vi "Plot Editor.vi"(6 "Original Plot Idx":i32=-1, 7 "Original Graph Name":string, 8 "Error In":errorcluster, 9 "Plot Style in":T2={"Plot Index"=0, "Plot.Bar Plot Style"=0, "Plot.DigitalLineStyle"=1, "Plot.TransitionLocation"=2, "Plot.Transition Type"=0, "Plot.Fill To"=-1, "Plot.Fill/Pt. Color"=16777222, "Plot.Label Format"=3, "Plot.Line Style"=0, "Plot.Line Width"=1, "Plot.Plot Color"=16777222, "Plot.Plot Interpolation"=2, "Plot.Plot Name"="", "Plot.Point Style"=0, "Plot.Visible?"=TRUE, "Plot.XScaleIdx"=0, "Plot.YScaleIdx"=0, "Plot.Anti-aliased"=TRUE}, 10 "Plot in":T3, 11 "Original Graph Refnum":T1) -> (0 "Error Out":errorcluster, 1 "Plot Style out":T2, 2 "Plot out":T3)   [LabVIEW 2019, in "Plot Editor.lvlib"]
uses:
  Plot Editor.lvlib
  XY Graph Plot Properties.ctl
  XY Plot Data.ctl
  XY Graph Refnum.ctl
  Plot Editor Q [Element].ctl
  Plot Editor Q [Event] List.ctl
  Plot Editor Internal Variables.ctl
  <vilib>/Utility/error.llb/DialogType.ctl
  <vilib>/Utility/miscctls.llb/LVPoint32TypeDef.ctl
  XY Graph Add-Ons.lvlib
  Notebook.lvlib
  Define Ramp Array Dialog.vi
  Rich Text Box.lvlib
  Variant to Data.lvlib
panel:
  in  "X Array":dbl[](array[numeric])
  in  "Copy":bool
  in  "Cancel":bool
  out "Error":errorcluster
  in  "Reset Style":bool
  out "Y Array Size":i32
  in  "Cancel Data Edit":bool
  in  "OK":bool
  out "X Array Size":i32
  in  "Y Array":dbl[](array[numeric]) caption="X Array"
  out "Plot Preview":cluster{"X Array":dbl[], "Y Array":dbl[]}[](graph)
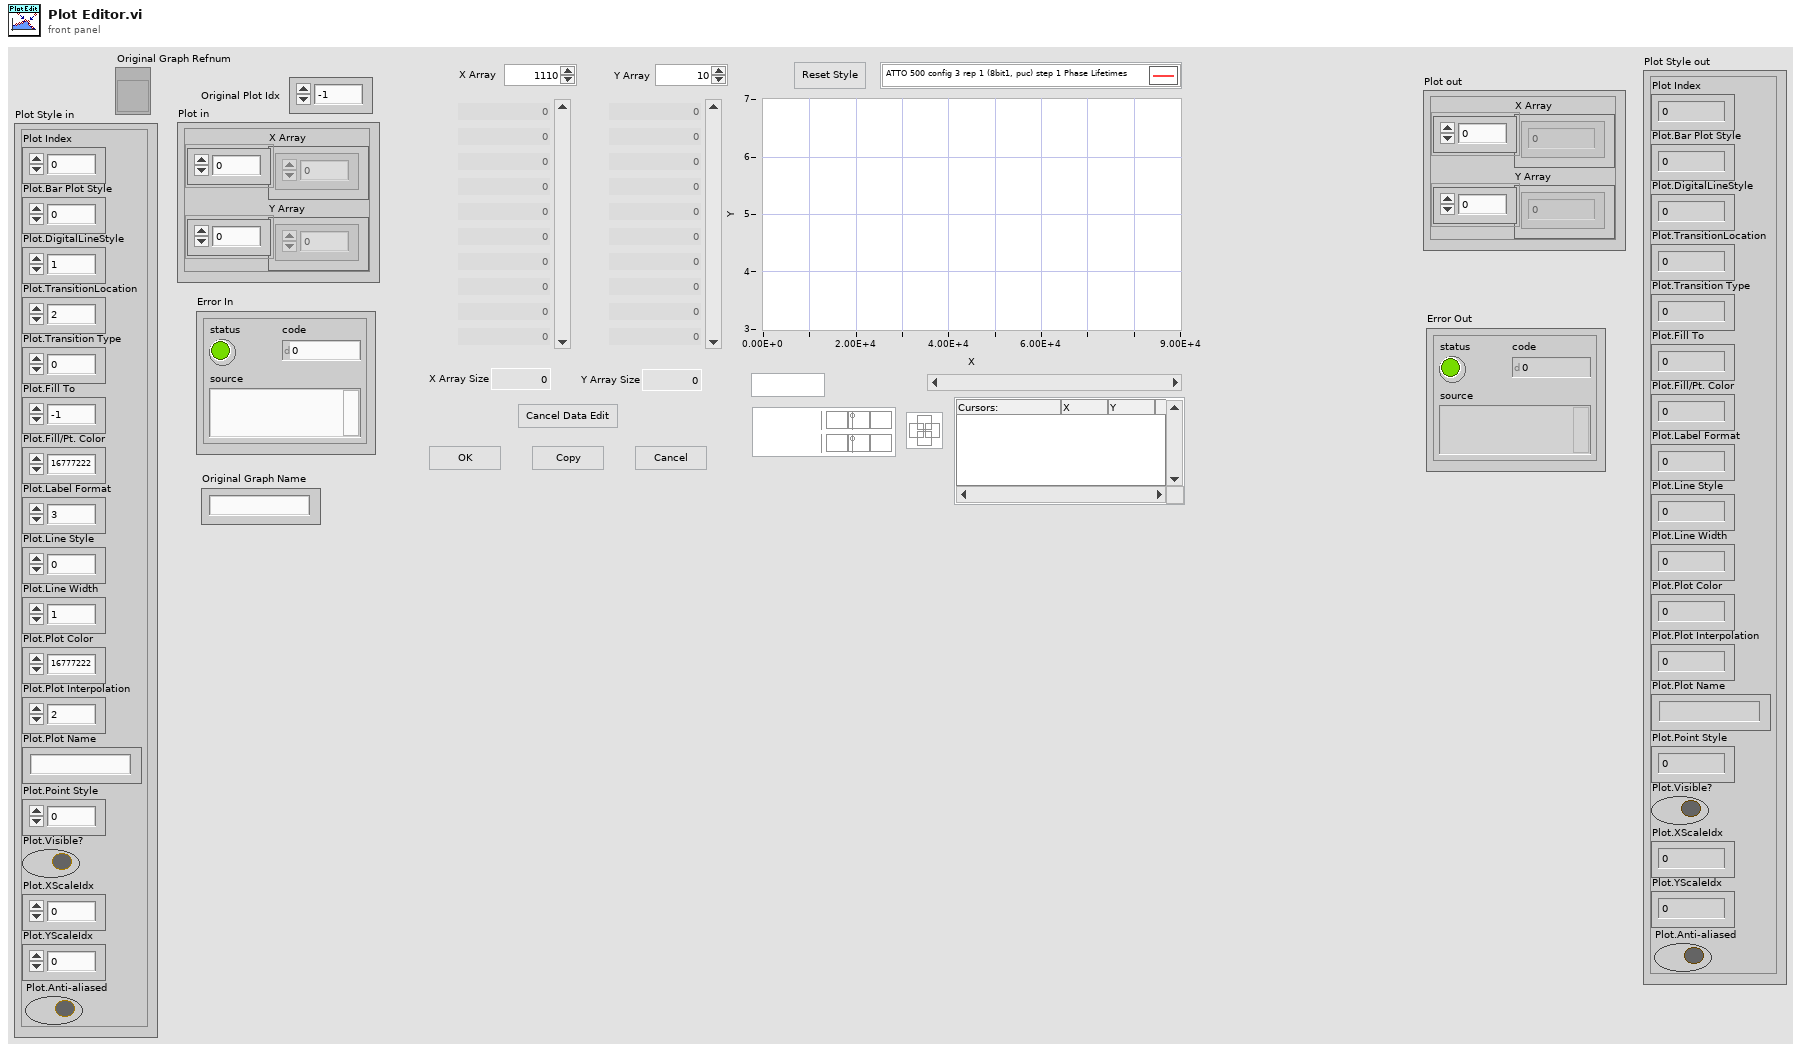
[diagram p1: front panel]
types:
  T1 = typedef "XY Graph Add-Ons.lvlib/XY Graph Refnum.ctl" = refnum<vi>
  T2 = typedef "XY Graph Plot Properties.ctl" = cluster{"Plot Index":i32, "Plot.Bar Plot Style":u8, "Plot.DigitalLineStyle":u8, "Plot.TransitionLocation":u8, "Plot.Transition Type":u8, "Plot.Fill To":i16, "Plot.Fill/Pt. Color":u32, "Plot.Label Format":u8, "Plot.Line Style":u8, "Plot.Line Width":u8, "Plot.Plot Color":u32, "Plot.Plot Interpolation":u8, "Plot.Plot Name":string, "Plot.Point Style":u8, "Plot.Visible?":bool, "Plot.XScaleIdx":u32, "Plot.YScaleIdx":u32, "Plot.Anti-aliased":bool}
  T3 = typedef "XY Plot Data.ctl" = cluster{"X Array":dbl[], "Y Array":dbl[]}
  T4 = typedef "Plot Editor.lvlib/Plot Editor Q [Element].ctl" = cluster{"Plot Editor Q Event":T5, "Data":variant}
  T5 = typedef "Plot Editor.lvlib/Plot Editor Q [Event] List.ctl" = enum16{"Idle", "Initialization", "Controls >> Store", "Store >> Plot", "Update Plot Style", "Check Data Array Alignment", "Reset Data", "Reset Style", "Accept & Quit", "Copy & Quit", "Save Plot", "Load Plot", "Remove out-of-bound Values", "Delete Element", "Insert Element Before", "Insert Element After", "Update output string", "Remove NaN-containing Pairs", "Fill Array with Ramp", "Quit"}
  T6 = typedef "Plot Editor.lvlib/Plot Editor Internal Variables.ctl" = cluster{"X Array":dbl[], "Y Array":dbl[], "XY Plot Properties":T2, "X Array Index Values":u32[], "Y Array Index Values":u32[], "Original XY Plot Properties":T2, "Original X Array":dbl[], "Original Y Array":dbl[], "VI title suffix":string, "Refnum based call":bool}
  T7 = typedef "LVPoint32TypeDef.ctl" = cluster{"Horizontal":i32, "Vertical":i32}
  T8 = typedef "Rich Text Box.lvlib/Text Formatting.ctl" = cluster{"Font":string, "Text Color":T9, "Text Background Color":T9, "Text Style":enum16{"Regular", "Bold", "Italic", "Underline", "Strikeout"}, "Font Size (Points)":dbl, "Text Alignment":i32}
  T9 = typedef "Rich Text Box.lvlib/Text Colors.ctl" = enum16{"Unchanged", "Black", "Blue", "Gray", "Green", "Red", "White"}
  T10 = typedef "DialogType.ctl" = u16
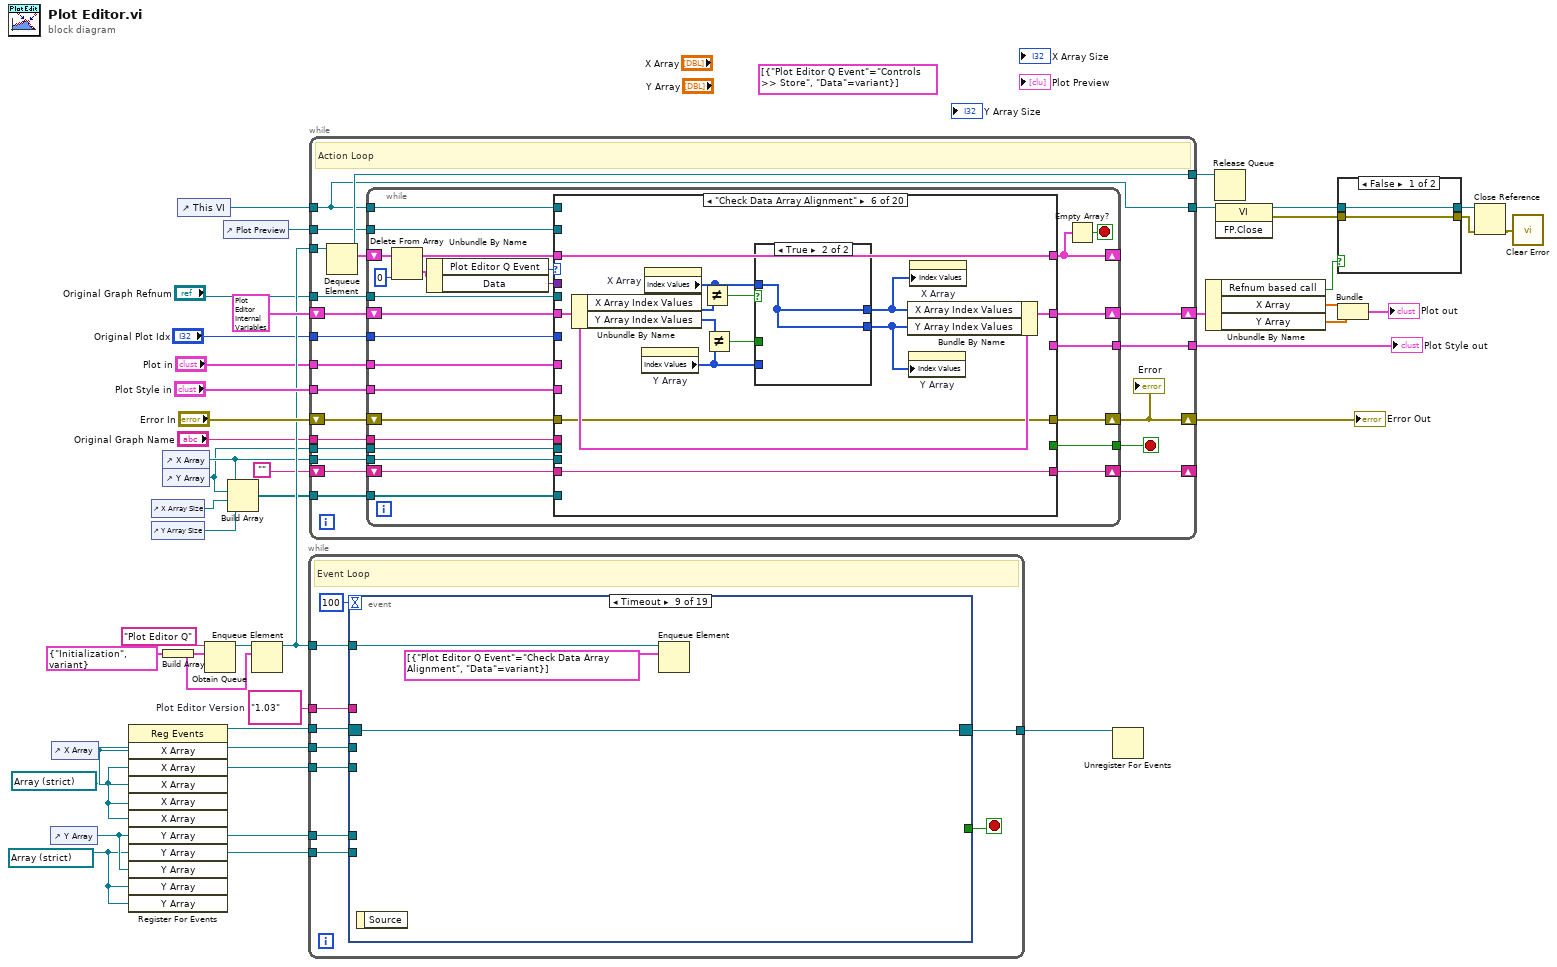
[diagram p0: block diagram]
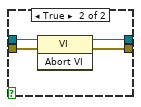
[diagram p2: hidden frame]
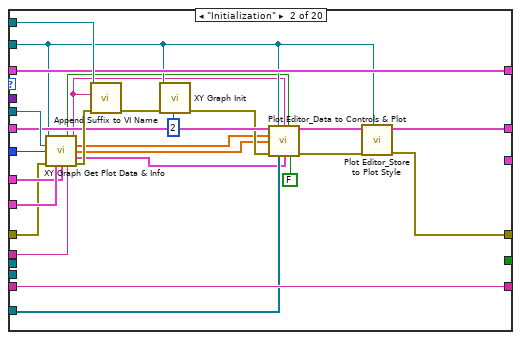
[diagram p4: hidden frame]
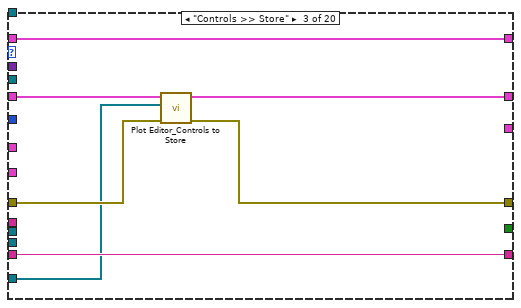
[diagram p5: hidden frame]
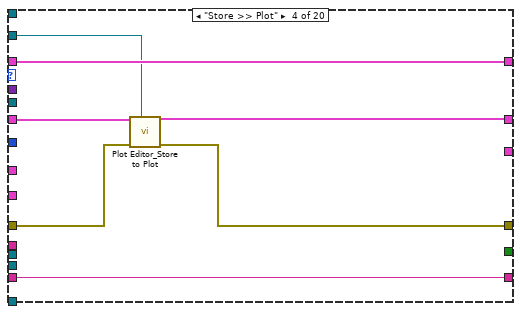
[diagram p6: hidden frame]
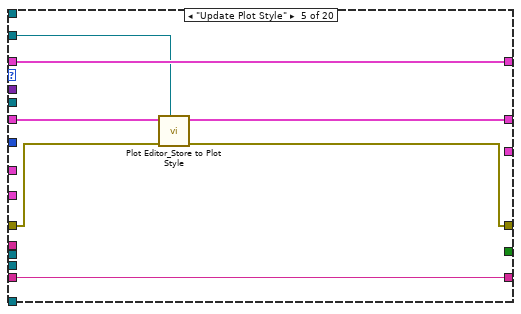
[diagram p7: hidden frame]
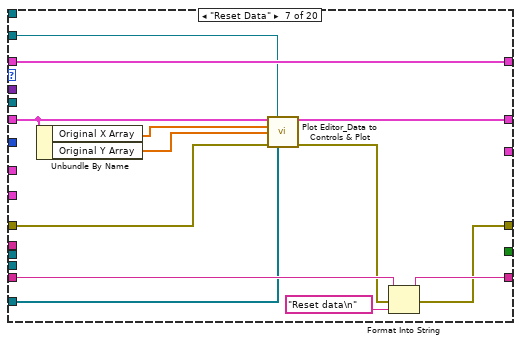
[diagram p10: hidden frame]
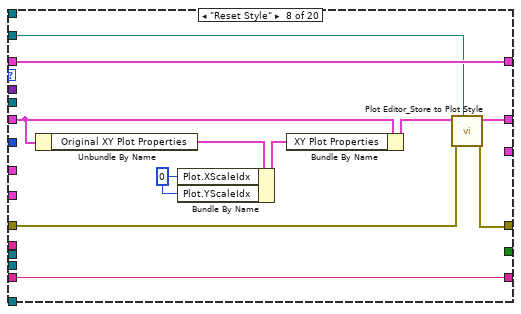
[diagram p11: hidden frame]
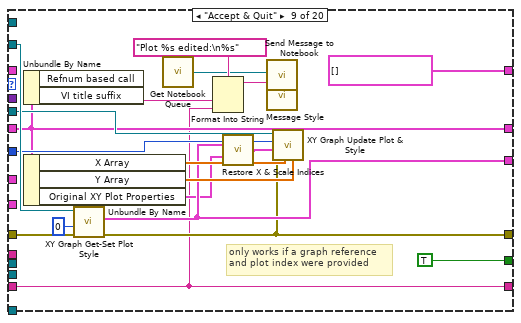
[diagram p12: hidden frame]
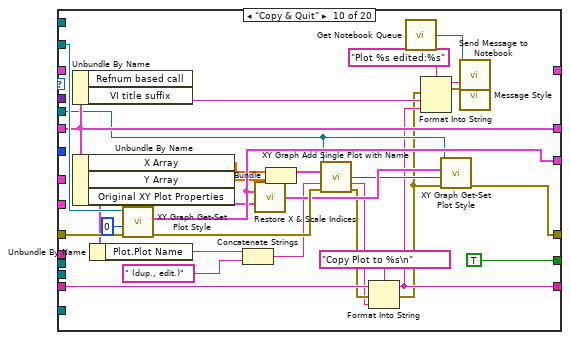
[diagram p13: hidden frame]
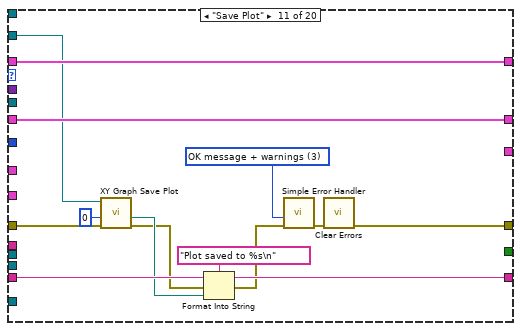
[diagram p14: hidden frame]
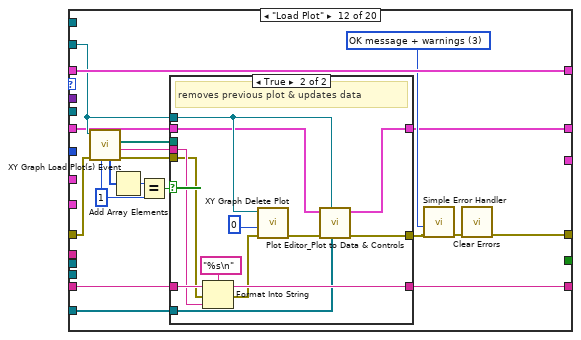
[diagram p15: hidden frame]
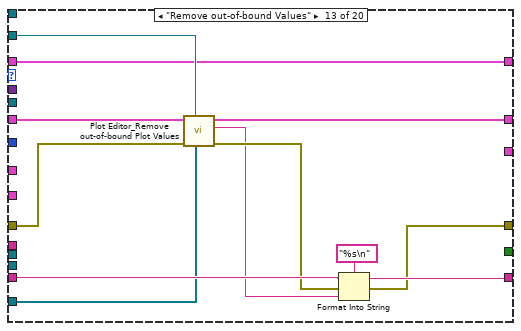
[diagram p17: hidden frame]
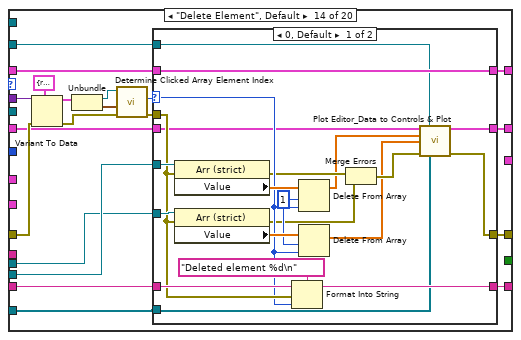
[diagram p18: hidden frame]
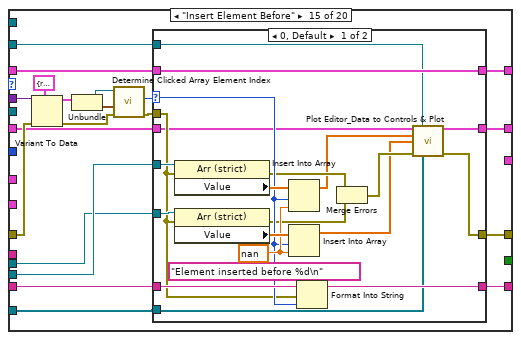
[diagram p20: hidden frame]
diagram:
  w2 = refnum<vi> refnum ("Y Array")
  w1 = refnum<vi> refnum ("X Array")
  (unwired) T4[] [{"Plot Editor Q Event"=enum."Controls >> Store", "Data"=variant}] ("array")
  w25 = "1.03"  # Plot Editor Version
  n1 = control-ref of="Y Array"() -> (w3:refnum<vi>)
  n2 = control-ref of="X Array"() -> (w4:refnum<vi>)
  n3 = register-events(w4, w1, w4, w1, w1, w3, w2, w3, w2, w2) -> (reference out=w24:refnum<event-registration>)  [unwired: 2 in, 1 out]
  n4 = control-ref of="X Array Size"() -> (w7:refnum<vi>)
  n5 = control-ref of="Y Array Size"() -> (w6:refnum<vi>)
  n6 = control-ref of="X Array"() -> (w9:refnum<vi>)
  n7 = control-ref of="Y Array"() -> (w8:refnum<vi>)
  n8 = Build Array(T4 {"Plot Editor Q Event"=enum."Initialization", "Data"=variant} ("Plot Editor Q Element")) -> (w26:T4[])
  n9 = control-ref of="This VI"() -> (w16:refnum<vi>)
  n10 = Obtain Queue(name (unnamed)="Plot Editor Q", element data type=w26) -> (queue out=w39:refnum<queue>)  [unwired: 3 in, 2 out]
  n11 = control-ref of="Plot Preview"() -> (w34:refnum<vi>)
  n12 = Build Array(w9, w8, w7, w6) -> (w5:refnum<vi>[])
  n13 = Enqueue Element(queue=w39, element=w26) -> (queue out=w27:refnum<queue>)  [unwired: 2 in, 2 out]
  n14 = while {
    tunnel: w27 -> [w50]
    tunnel: w25 -> [w49]
    tunnel: w24 -> [w48]
    tunnel: w4 -> [w47]
    tunnel: w3 -> [w46]
    tunnel: [w45] -> w23
    tunnel: w1 -> [w44]
    tunnel: w2 -> [w43]
    stop <- w51 stop-if-true
    # "Event Loop"
    n15 = event shown="[8] Timeout" {
      selector: w48 -> [_ _ _ _ _ w157 w161 w164 w167 w173 w179 w183 w188 _ _ _ _ _ _]
      dyn-events: [_ _ _ _ _ w156 w160 w164 w167 w172 w178 w182 w187 _ _ _ _ _ _] -> w45
      timeout: 100 -> [_ _ _ _ _ _ _ _ _ _ _ _ _ _ _ _ _ _ _]
      tunnel: [w54 w56 _ _ _ _ _ _ _ _ _ _ _ _ _ _ TRUE ("Discard?") TRUE ("Discard?") TRUE ("Discard?")] -> w51
      tunnel: w50 -> [w53 w57 w91 w122 w146 _ _ w163 w166 w169 w174 _ _ w198 w200 w202 w205 w208 w211]
      tunnel: w49 -> [_ w55 _ _ _ _ _ _ _ _ _ _ _ _ _ _ _ _ _]
      tunnel: w47 -> [_ _ _ _ _ w155 _ _ _ w171 _ w181 w186 _ _ _ _ _ _]
      tunnel: w46 -> [_ _ _ _ _ _ w159 _ _ _ w176 _ w185 _ _ _ _ _ _]
      tunnel: w44 -> [_ _ _ _ _ w154 _ _ _ w170 _ w180 _ _ _ _ _ _ _]
      tunnel: w43 -> [_ _ _ _ _ _ w158 _ _ _ w177 _ w184 _ _ _ _ _ _]
      event Panel Close? {
        w54 = TRUE ("Discard?")
        n16 = event-data() -> ()  [unwired: 1 in, 1 out]
        n17 = Enqueue Element(queue=w53, element=T4[] [{"Plot Editor Q Event"=enum."Quit", "Data"=variant}]) -> ()  [unwired: 2 in, 3 out]
        n18 = event-data("Discard?"=w54) -> ()  [unwired: 1 in, 1 out]
      }
      event Menu Selection (User) {
        n19 = event-data() -> ("ItemTag"=w58:string)  [unwired: 1 in]
        n20 = case shown="\"About...\"" w58 {
          tunnel: w57 -> [_ w60 w62 w66 w79 _]
          tunnel: [_ _ _ w63 _ _] -> w56
          tunnel: w55 -> [_ _ _ _ _ w84]
          frame "", Default {
          }
          frame "Save Plot" {
            n21 = Enqueue Element(queue=w60, element=T4[] [{"Plot Editor Q Event"=enum."Save Plot", "Data"=variant}]) -> ()  [unwired: 2 in, 3 out]
          }
          frame "Load Plot" {
            n22 = Enqueue Element(queue=w62, element=T4[] [{"Plot Editor Q Event"=enum."Load Plot", "Data"=variant}]) -> ()  [unwired: 2 in, 3 out]
          }
          frame "Quit" {
            n23 = call "Two Buttons Dialog Window.vi"("OK Button Text"="Accept & Quit" ("T button name (\"OK\")"), "Message"="Are you sure you want to quit Plot Editor?\nQuitting will save the current changes and return to the original graph." ("message")) -> ("OK?"=w63:bool)  [unwired: 1 in]
            n24 = case shown="True" w63 {
              tunnel: w66 -> [_ w68]
              frame False {
              }
              frame True {
                n25 = Enqueue Element(queue=w68, element=T4[] [{"Plot Editor Q Event"=enum."Accept & Quit", "Data"=variant}]) -> ()  [unwired: 2 in, 3 out]
              }
            }
          }
          frame "Paste Data from Clipboard" {
            w70 = "\n"
            n26 = invoke class="App" method="Clipboard.Read"() -> ("Read Clipbrd"=w76:string)  [unwired: 3 in, 2 out]
            n27 = call <userlib>:"String to 1D Array__ogtk.vi"("delimiter (Tab)"=w70, "string"=w76) -> ("Array of Strings"=w75:string[])  [unwired: 9 in]
            n28 = Delete From Array(array=w75, length=1, index=0) -> (array with subset deleted=w72:string[])  [unwired: 1 out]
            n29 = call <userlib>:"1D Array to String__ogtk.vi"("delimiter (Tab)"=w70, "Array of Strings"=w72) -> ("delimited string"=w71:string)  [unwired: 9 in]
            n30 = Spreadsheet String To Array(format string="%#g", spreadsheet string=w71) -> (array=w82:dbl[][])  [unwired: 2 in]
            n31 = Transpose 2D Array(2D array=w82) -> (transposed array=w69:dbl[][])
            n32 = Enqueue Element(queue=w79, element=T4[] [{"Plot Editor Q Event"=enum."Controls >> Store", "Data"=variant}, {"Plot Editor Q Event"=enum."Store >> Plot", "Data"=variant}]) -> ()  [unwired: 2 in, 3 out]
            n33 = Index Array(array=w69) -> (element #1=w81:dbl[], element #2=w80:dbl[])  [unwired: 4 in]
            n34 = local write "X Array"(w81) -> ()
            n35 = local write "Y Array"(w80) -> ()
          }
          frame "About..." {
            n36 = Format Into String(format string="                                      Plot Editor\n                                      version %s\n\n                              Author: X. Michalet\n(c) 2017-2020 The Regents of the  University of California" ("message"), w84) -> (resulting string=w83:string)  [unwired: 2 in, 1 out]
            n37 = One Button Dialog(message=w83) -> ()  [unwired: 1 in, 1 out]
          }
        }
      }
      event "X Array": Shortcut Menu Selection (User) {
        n38 = event-data() -> ("ItemTag"=w92:string, "CtlRef"=w89:refnum<vi>, "Coords"=w88:T7)  [unwired: 1 in]
        n39 = case shown="\"Remove NaN-containing Pairs\"" w92 {
          tunnel: [w93 w99 w105 w111 w114 w116] -> w90
          tunnel: w89 -> [_ w98 w104 w110 _ _]
          tunnel: w88 -> [_ w97 w103 w109 _ _]
          frame "", Default {
            n40 = Build Array(T4 {"Plot Editor Q Event"=enum."Idle", "Data"=variant} ("Plot Editor Q Element")) -> (w93:T4[])
          }
          frame "Delete Element" {
            n41 = Bundle("CtlRef"=w98, "Coords"=w97) -> (w95:cluster{"CtlRef":refnum<vi>, "Coords":T7})  [unwired: 1 in]
            n42 = Bundle By Name(cluster=T4 {"Plot Editor Q Event"=enum."Delete Element", "Data"=variant} ("Plot Editor Q Element"), "Data"=w95) -> (w96:T4)
            n43 = Build Array(w96) -> (w99:T4[])
          }
          frame "Insert Element Before" {
            n44 = Bundle("CtlRef"=w104, "Coords"=w103) -> (w101:cluster{"CtlRef":refnum<vi>, "Coords":T7})  [unwired: 1 in]
            n45 = Bundle By Name(cluster=T4 {"Plot Editor Q Event"=enum."Insert Element Before", "Data"=variant} ("Plot Editor Q Element"), "Data"=w101) -> (w102:T4)
            n46 = Build Array(w102) -> (w105:T4[])
          }
          frame "Insert Element After" {
            n47 = Bundle("CtlRef"=w110, "Coords"=w109) -> (w107:cluster{"CtlRef":refnum<vi>, "Coords":T7})  [unwired: 1 in]
            n48 = Bundle By Name(cluster=T4 {"Plot Editor Q Event"=enum."Insert Element After", "Data"=variant} ("Plot Editor Q Element"), "Data"=w107) -> (w108:T4)
            n49 = Build Array(w108) -> (w111:T4[])
          }
          frame "Fill Array with Ramp" {
            n50 = Build Array(T4 {"Plot Editor Q Event"=enum."Fill Array with Ramp", "Data"=variant} ("Plot Editor Q Element")) -> (w114:T4[])
          }
          frame "Remove NaN-containing Pairs" {
            n51 = Build Array(T4 {"Plot Editor Q Event"=enum."Remove NaN-containing Pairs", "Data"=variant} ("Plot Editor Q Element")) -> (w116:T4[])
          }
        }
        n52 = Build Array (concatenate)(w90, T4[] [{"Plot Editor Q Event"=enum."Controls >> Store", "Data"=variant}, {"Plot Editor Q Event"=enum."Store >> Plot", "Data"=variant}] ("array")) -> (w87:T4[])
        n53 = Enqueue Element(queue=w91, element=w87) -> ()  [unwired: 2 in, 3 out]
      }
      event "Y Array": Shortcut Menu Selection (User) {
        n54 = event-data() -> ("ItemTag"=w123:string, "CtlRef"=w121:refnum<vi>, "Coords"=w120:T7)  [unwired: 1 in]
        n55 = case shown="\"Remove NaN-containing Pairs\"" w123 {
          tunnel: [w124 w128 w134 w140 w145] -> w119
          tunnel: w121 -> [_ w127 w133 w139 _]
          tunnel: w120 -> [_ w126 w132 w138 _]
          frame "", Default {
            n56 = Build Array(T4 {"Plot Editor Q Event"=enum."Idle", "Data"=variant} ("Plot Editor Q Element")) -> (w124:T4[])
          }
          frame "Delete Element" {
            n57 = Bundle("CtlRef"=w127, "Coords"=w126) -> (w130:cluster{"CtlRef":refnum<vi>, "Coords":T7})  [unwired: 1 in]
            n58 = Bundle By Name(cluster=T4 {"Plot Editor Q Event"=enum."Delete Element", "Data"=variant} ("Plot Editor Q Element"), "Data"=w130) -> (w131:T4)
            n59 = Build Array(w131) -> (w128:T4[])
          }
          frame "Insert Element Before" {
            n60 = Bundle("CtlRef"=w133, "Coords"=w132) -> (w136:cluster{"CtlRef":refnum<vi>, "Coords":T7})  [unwired: 1 in]
            n61 = Bundle By Name(cluster=T4 {"Plot Editor Q Event"=enum."Insert Element Before", "Data"=variant} ("Plot Editor Q Element"), "Data"=w136) -> (w137:T4)
            n62 = Build Array(w137) -> (w134:T4[])
          }
          frame "Insert Element After" {
            n63 = Bundle("CtlRef"=w139, "Coords"=w138) -> (w142:cluster{"CtlRef":refnum<vi>, "Coords":T7})  [unwired: 1 in]
            n64 = Bundle By Name(cluster=T4 {"Plot Editor Q Event"=enum."Insert Element After", "Data"=variant} ("Plot Editor Q Element"), "Data"=w142) -> (w143:T4)
            n65 = Build Array(w143) -> (w140:T4[])
          }
          frame "Remove NaN-containing Pairs" {
            n66 = Build Array(T4 {"Plot Editor Q Event"=enum."Remove NaN-containing Pairs", "Data"=variant} ("Plot Editor Q Element")) -> (w145:T4[])
          }
        }
        n67 = Build Array (concatenate)(w119, T4[] [{"Plot Editor Q Event"=enum."Controls >> Store", "Data"=variant}, {"Plot Editor Q Event"=enum."Store >> Plot", "Data"=variant}] ("array")) -> (w118:T4[])
        n68 = Enqueue Element(queue=w122, element=w118) -> ()  [unwired: 2 in, 3 out]
      }
      event "Plot Preview": Shortcut Menu Selection (User) {
        n69 = event-data() -> ("ItemTag"=w147:string)  [unwired: 1 in, 1 out]
        n70 = case shown="\"Remove out-of-bound Values\"" w147 {
          tunnel: w146 -> [_ w149 w151 w153]
          frame "", Default {
          }
          frame "Save Plot" {
            n71 = Enqueue Element(queue=w149, element=T4[] [{"Plot Editor Q Event"=enum."Save Plot", "Data"=variant}]) -> ()  [unwired: 2 in, 3 out]
          }
          frame "Load Plot" {
            n72 = Enqueue Element(queue=w151, element=T4[] [{"Plot Editor Q Event"=enum."Load Plot", "Data"=variant}]) -> ()  [unwired: 2 in, 3 out]
          }
          frame "Remove out-of-bound Values" {
            n73 = Enqueue Element(queue=w153, element=T4[] [{"Plot Editor Q Event"=enum."Remove out-of-bound Values", "Data"=variant}]) -> ()  [unwired: 2 in, 3 out]
          }
        }
      }
      event Mouse Down {
        n74 = event-data() -> ()  [unwired: 1 in, 1 out]
        n75 = register-events(reference=w157, w154, w155, w155, w155) -> (reference out=w156:refnum<event-registration>)  [unwired: 7 in, 1 out]
      }
      event Mouse Down {
        n76 = event-data() -> ()  [unwired: 1 in, 1 out]
        n77 = register-events(reference=w161, w158, w159, w159, w159) -> (reference out=w160:refnum<event-registration>)  [unwired: 7 in, 1 out]
      }
      event Mouse Move; Mouse Wheel {
        n78 = event-data() -> ()  [unwired: 1 in, 1 out]
        n79 = Enqueue Element(queue=w163, element=T4[] [{"Plot Editor Q Event"=enum."Check Data Array Alignment", "Data"=variant}]) -> ()  [unwired: 2 in, 3 out]
      }
      event Timeout {
        n80 = event-data() -> ()  [unwired: 1 in, 1 out]
        n81 = Enqueue Element(queue=w166, element=T4[] [{"Plot Editor Q Event"=enum."Check Data Array Alignment", "Data"=variant}]) -> ()  [unwired: 2 in, 3 out]
      }
      event Mouse Up {
        n82 = event-data() -> ()  [unwired: 1 in, 1 out]
        n83 = register-events(reference=w173, w171, w170, w170) -> (reference out=w172:refnum<event-registration>)  [unwired: 8 in, 1 out]
        n84 = Enqueue Element(queue=w169, element=T4[] [{"Plot Editor Q Event"=enum."Check Data Array Alignment", "Data"=variant}]) -> ()  [unwired: 2 in, 3 out]
      }
      event Mouse Up {
        n85 = event-data() -> ()  [unwired: 1 in, 1 out]
        n86 = register-events(reference=w179, w176, w177, w177) -> (reference out=w178:refnum<event-registration>)  [unwired: 8 in, 1 out]
        n87 = Enqueue Element(queue=w174, element=T4[] [{"Plot Editor Q Event"=enum."Check Data Array Alignment", "Data"=variant}]) -> ()  [unwired: 2 in, 3 out]
      }
      event Mouse Leave {
        n88 = event-data() -> ()  [unwired: 1 in, 1 out]
        n89 = register-events(reference=w183, w181, w180, w180, w180) -> (reference out=w182:refnum<event-registration>)  [unwired: 7 in, 1 out]
      }
      event Mouse Leave {
        n90 = event-data() -> ()  [unwired: 1 in, 1 out]
        n91 = register-events(reference=w188, w186, w185, w184, w184, w184) -> (reference out=w187:refnum<event-registration>)  [unwired: 6 in, 1 out]
      }
      event "X Array", "Y Array": Value Change {
        n92 = event-data() -> ("CtlRef"=w193:refnum<vi>)  [unwired: 1 in]
        n93 = property class="Arr (strict)"(reference=w193) -> (error out=w190:errorcluster, "Label.Text"=w191:string)  [unwired: 1 in, 1 out]
        n94 = Format Into String(format string="User added %s data", error in=w190, w191) -> (resulting string=w189:string)  [unwired: 1 in, 1 out]
        n95 = Bundle By Name(cluster=T4 {"Plot Editor Q Event"=enum."Update output string", "Data"=variant} ("Plot Editor Q Element"), "Data"=w189) -> (w194:T4)
        n96 = Build Array (concatenate)(T4[] [{"Plot Editor Q Event"=enum."Controls >> Store", "Data"=variant}, {"Plot Editor Q Event"=enum."Store >> Plot", "Data"=variant}, {"Plot Editor Q Event"=enum."Check Data Array Alignment", "Data"=variant}] ("element"), w194) -> (w196:T4[])
        n97 = Enqueue Element(queue=w198, element=w196) -> ()  [unwired: 2 in, 3 out]
      }
      event "Reset Style": Value Change {
        n98 = event-data() -> ()  [unwired: 1 in, 1 out]
        n99 = Enqueue Element(queue=w200, element=T4[] [{"Plot Editor Q Event"=enum."Reset Style", "Data"=variant}]) -> ()  [unwired: 2 in, 3 out]
      }
      event "Cancel Data Edit": Value Change {
        n100 = event-data() -> ()  [unwired: 1 in, 1 out]
        n101 = Enqueue Element(queue=w202, element=T4[] [{"Plot Editor Q Event"=enum."Reset Data", "Data"=variant}]) -> ()  [unwired: 2 in, 3 out]
      }
      event "OK": Value Change {
        n102 = event-data() -> ()  [unwired: 1 in, 1 out]
        n103 = Enqueue Element(queue=w205, element=T4[] [{"Plot Editor Q Event"=enum."Accept & Quit", "Data"=variant}]) -> ()  [unwired: 2 in, 3 out]
      }
      event "Copy": Value Change {
        n104 = event-data() -> ()  [unwired: 1 in, 1 out]
        n105 = Enqueue Element(queue=w208, element=T4[] [{"Plot Editor Q Event"=enum."Copy & Quit", "Data"=variant}]) -> ()  [unwired: 2 in, 3 out]
      }
      event "Cancel": Value Change {
        n106 = event-data() -> ()  [unwired: 1 in, 1 out]
        n107 = Enqueue Element(queue=w211, element=T4[] [{"Plot Editor Q Event"=enum."Quit", "Data"=variant}]) -> ()  [unwired: 2 in, 3 out]
      }
    }
  }
  n108 = while {
    tunnel: w27 -> [w232]
    tunnel: [w229] -> w38
    shift-right: [w226] -> w32
    shift-left: T6 {"X Array"=[], "Y Array"=[], "XY Plot Properties"={"Plot Index"=0, "Plot.Bar Plot Style"=0, "Plot.DigitalLineStyle"=0, "Plot.TransitionLocation"=0, "Plot.Transition Type"=0, "Plot.Fill To"=-1, "Plot.Fill/Pt. Color"=0, "Plot.Label Format"=0, "Plot.Line Style"=0, "Plot.Line Width"=0, "Plot.Plot Color"=0, "Plot.Plot Interpolation"=0, "Plot.Plot Name"="Plot", "Plot.Point Style"=0, "Plot.Visible?"=FALSE, "Plot.XScaleIdx"=0, "Plot.YScaleIdx"=0, "Plot.Anti-aliased"=FALSE}, "X Array Index Values"=[], "Y Array Index Values"=[], "Original XY Plot Properties"={"Plot Index"=0, "Plot.Bar Plot Style"=0, "Plot.DigitalLineStyle"=0, "Plot.TransitionLocation"=0, "Plot.Transition Type"=0, "Plot.Fill To"=0, "Plot.Fill/Pt. Color"=0, "Plot.Label Format"=0, "Plot.Line Style"=0, "Plot.Line Width"=0, "Plot.Plot Color"=0, "Plot.Plot Interpolation"=0, "Plot.Plot Name"="", "Plot.Point Style"=0, "Plot.Visible?"=FALSE, "Plot.XScaleIdx"=0, "Plot.YScaleIdx"=0, "Plot.Anti-aliased"=FALSE}, "Original X Array"=[], "Original Y Array"=[], "VI title suffix"="", "Refnum based call"=FALSE} ("Plot Editor Internal Data") -> [w228]
    shift-right: [w217] -> w33
    shift-left: "Error In" -> [w225]
    tunnel: "Plot Style in" -> [w227]
    tunnel: w34 -> [w224]
    tunnel: [w223] -> w28
    tunnel: "Original Graph Refnum" -> [w222]
    tunnel: "Original Plot Idx" -> [w221]
    tunnel: "Plot in" -> [w220]
    tunnel: "Original Graph Name" -> [w219]
    tunnel: w16 -> [w218]
    tunnel: [w218] -> w18
    shift-right: [w215] -> _
    shift-left: "" -> [w216]
    tunnel: w9 -> [w214]
    tunnel: w8 -> [w213]
    tunnel: w5 -> [w212]
    stop <- w230 stop-if-true
    # "Action Loop"
    n109 = Dequeue Element(queue=w232) -> (queue out=w229:refnum<queue>, element=w231:T4[])  [unwired: 2 in, 2 out]
    n110 = while {
      tunnel: [w258] -> w230
      shift-right: [w254] -> _
      shift-left: w231 -> [w257]
      tunnel: w227 -> [w251]
      tunnel: w224 -> [w233]
      shift-right: [w250] -> w226
      shift-left: w228 -> [w252]
      shift-right: [w246] -> w217
      shift-left: w225 -> [w247]
      tunnel: [w245] -> w223
      tunnel: w222 -> [w244]
      tunnel: w221 -> [w243]
      tunnel: w220 -> [w242]
      tunnel: w219 -> [w241]
      tunnel: w218 -> [w240]
      shift-right: [w237] -> w215
      shift-left: w216 -> [w238]
      tunnel: w214 -> [w236]
      tunnel: w213 -> [w235]
      tunnel: w212 -> [w234]
      stop <- w253 stop-if-true
      n111 = Delete From Array(array=w257, index=0) -> (deleted portion=w249:T4, array with subset deleted=w255:T4[])  [unwired: 1 in]
      n112 = Unbundle By Name(w249) -> ("Plot Editor Q Event"=w248:T5, "Data"=w239:variant)
      n113 = case shown="\"Check Data Array Alignment\"" w248 {
        tunnel: [_ _ _ _ _ _ _ _ TRUE TRUE _ _ _ _ _ _ _ _ _ TRUE] -> w258
        tunnel: w255 -> [w262 w277 w295 w302 w309 w316 w341 w355 _ _ w419 w438 w458 w474 w519 w564 w611 w616 w649 _]
        tunnel: [w262 w277 w295 w302 w309 w316 w341 w355 T4[] [] _ w419 w438 w458 w473 w518 w563 w611 w616 w646 T4[] []] -> w254
        tunnel: w252 -> [w260 w274 w293 w298 w305 w318 w338 w354 w368 w403 w418 w427 w457 w470 w515 w560 w603 w615 w656 w685]
        tunnel: w251 -> [_ w286 _ _ _ _ _ _ _ _ _ _ _ _ _ _ _ _ _ _]
        tunnel: [w260 w275 w292 w299 w304 w317 w337 w348 w368 w403 w418 w426 w456 w467 w514 w559 w603 w613 w655 w686] -> w250
        tunnel: w247 -> [w261 w284 w290 w296 w308 w313 w336 w347 w366 w401 w416 w437 w466 w471 w517 w562 w605 w621 w654 _]
        tunnel: [w261 w276 w291 w297 w307 w313 w340 w346 w364 w397 w413 w434 w461 w472 w516 w561 w606 w619 w647 _] -> w246
        tunnel: [_ _ _ _ _ _ _ _ w365 w400 _ _ _ _ _ _ _ _ _ w682] -> w245
        tunnel: w244 -> [_ w288 _ _ _ _ _ _ w372 w396 _ _ _ _ _ _ _ _ _ _]
        tunnel: w243 -> [_ w287 _ _ _ _ _ _ w371 _ _ _ _ _ _ _ _ _ _ _]
        tunnel: w242 -> [_ w285 _ _ _ _ _ _ _ _ _ _ _ _ _ _ _ _ _ _]
        tunnel: w241 -> [_ w283 _ _ _ _ _ _ _ _ _ _ _ _ _ _ _ _ _ _]
        tunnel: w240 -> [_ w282 _ _ _ _ _ _ _ _ _ _ _ _ _ _ _ _ _ _]
        tunnel: w239 -> [_ _ _ _ _ _ _ _ _ _ _ _ _ w486 w531 w576 w610 w627 _ _]
        tunnel: w236 -> [_ _ _ _ _ _ _ _ _ _ _ _ _ w480 w525 w573 _ _ _ _]
        tunnel: w235 -> [_ _ _ _ _ _ _ _ _ _ _ _ _ w479 w524 w572 _ _ _ _]
        tunnel: w238 -> [w259 w279 w294 w301 w306 w312 w344 w350 w356 w386 w411 w424 w465 w476 w521 w566 w609 w623 w651 w680]
        tunnel: [w259 w279 w294 w301 w306 w312 w343 w350 w356 w379 w408 w423 w464 w475 w520 w565 w608 w622 w650 w680] -> w237
        tunnel: w234 -> [_ w269 w289 _ _ _ w332 _ _ _ _ w420 w455 w469 w512 w558 _ w614 w645 _]
        tunnel: w233 -> [_ w272 _ w300 w303 _ w333 w345 w374 w405 w417 w429 w460 w468 w513 w557 _ w612 w644 _]
        frame "Idle" {
        }
        frame "Initialization" {
          n114 = call "XY Graph Get Plot Data & Info.vi"("Destination Graph"=w272, "Original Graph"=w288, "Original Plot Idx"=w287, "Error In"=w284, "Plot Style in"=w286, "Plot in"=w285, "Graph Origin Name"=w283) -> ("Refnum based call"=w263:bool, "VI Title Suffix"=w264:string, "X Array"=w268:dbl[], "Y Array"=w267:dbl[], "Plot Style out"=w265:T2, "Error Out"=w281:errorcluster)  [unwired: 3 in]
          n115 = call "Append Suffix to VI Name.vi"("error in (no error)"=w281, "VI Title Suffix"=w264, "VI in"=w282) -> ("Error Out"=w278:errorcluster)  [unwired: 8 in]
          n116 = call "XY Graph Init.vi"("Max Legend Size (8)"=2 ("Plot.XScaleIdx"), "Error In"=w278, "XYGraph in"=w272) -> ("Error Out"=w271:errorcluster)  [unwired: 8 in]
          n117 = call "Plot Editor_Data to Controls & Plot.vi"("Plot Editor Internal Data"=w274, "XYGraph in"=w272, "VI Title Suffix"=w264, "Refnum based call"=w263, "X Array"=w268, "Y Array"=w267, "error in (no error)"=w271, "Control Refnums"=w269, "Plot Style"=w265, "Data only (T)"=FALSE) -> ("Plot Editor Internal Data"=w273:T6, "error out"=w270:errorcluster)  [unwired: 4 in]
          n118 = call "Plot Editor_Store to Plot Style.vi"("XYGraph in"=w272, "error in (no error)"=w270, "Plot Editor Internal Data"=w273) -> ("error out"=w276:errorcluster, "Plot Editor Internal Data (dup)"=w275:T6)  [unwired: 7 in]
        }
        frame "Controls >> Store" {
          n119 = call "Plot Editor_Controls to Store.vi"("Error In"=w290, "Control Refnums"=w289, "Plot Editor Internal Data in"=w293) -> ("Error Out"=w291:errorcluster, "Plot Editor Internal Data out"=w292:T6)  [unwired: 7 in]
        }
        frame "Store >> Plot" {
          n120 = call "Plot Editor_Store to Plot.vi"("XYGraph in"=w300, "Error In"=w296, "Plot Editor Internal Data"=w298) -> ("Error Out"=w297:errorcluster, "Plot Editor Internal Data (dup)"=w299:T6)  [unwired: 7 in]
        }
        frame "Update Plot Style" {
          n121 = call "Plot Editor_Store to Plot Style.vi"("XYGraph in"=w303, "error in (no error)"=w308, "Plot Editor Internal Data"=w305) -> ("error out"=w307:errorcluster, "Plot Editor Internal Data (dup)"=w304:T6)  [unwired: 7 in]
        }
        frame "Check Data Array Alignment" {
          n122 = Unbundle By Name(w318) -> ("X Array Index Values"=w322:u32[], "Y Array Index Values"=w321:u32[])
          n123 = property on="Y Array" class="Arr (strict)"() -> ("Index Values"=w314:u32[])  [unwired: 2 in, 2 out]
          n124 = property on="X Array" class="Arr (strict)"() -> ("Index Values"=w319:u32[])  [unwired: 2 in, 2 out]
          n125 = Not Equal?(x=w319, y=w322) -> (x != y?=w320:bool)
          n126 = Not Equal?(x=w321, y=w314) -> (x != y?=w315:bool)
          n127 = case shown="True" w320 {
            tunnel: w319 -> [w323 w331]
            tunnel: [w324 w331] -> w310
            tunnel: [w325 w331] -> w311
            tunnel: w315 -> [w327 _]
            tunnel: w314 -> [w326 _]
            frame False {
              n128 = case shown="False" w327 {
                tunnel: w326 -> [w328 w330]
                tunnel: [w329 w330] -> w325
                tunnel: [w328 w330] -> w324
                tunnel: w323 -> [w329 _]
                frame False {
                }
                frame True {
                }
              }
            }
            frame True {
            }
          }
          n129 = Bundle By Name(cluster=w318, "X Array Index Values"=w311, "Y Array Index Values"=w310) -> (w317:T6)
          n130 = property on="Y Array" class="Arr (strict)"("Index Values"=w310) -> ()  [unwired: 2 in, 2 out]
          n131 = property on="X Array" class="Arr (strict)"("Index Values"=w311) -> ()  [unwired: 2 in, 2 out]
        }
        frame "Reset Data" {
          n132 = Unbundle By Name(w338) -> ("Original X Array"=w339:dbl[], "Original Y Array"=w335:dbl[])
          n133 = call "Plot Editor_Data to Controls & Plot.vi"("Plot Editor Internal Data"=w338, "XYGraph in"=w333, "X Array"=w339, "Y Array"=w335, "error in (no error)"=w336, "Control Refnums"=w332) -> ("Plot Editor Internal Data"=w337:T6, "error out"=w334:errorcluster)  [unwired: 8 in]
          n134 = Format Into String(initial string=w344, error in=w334, "Reset data\n" ("format string")) -> (resulting string=w343:string, error out=w340:errorcluster)  [unwired: 1 in]
        }
        frame "Reset Style" {
          w351 = u32 0 ("Plot.XScaleIdx")
          n135 = Unbundle By Name(w354) -> ("Original XY Plot Properties"=w353:T2)
          n136 = Bundle By Name(cluster=w353, "Plot.XScaleIdx"=w351, "Plot.YScaleIdx"=w351) -> (w352:T2)
          n137 = Bundle By Name(cluster=w354, "XY Plot Properties"=w352) -> (w349:T6)
          n138 = call "Plot Editor_Store to Plot Style.vi"("XYGraph in"=w345, "error in (no error)"=w347, "Plot Editor Internal Data"=w349) -> ("error out"=w346:errorcluster, "Plot Editor Internal Data (dup)"=w348:T6)  [unwired: 7 in]
        }
        frame "Accept & Quit" {
          # "only works if a graph reference\nand plot index were provided"
          n139 = Unbundle By Name(w368) -> ("VI title suffix"=w367:string)  [unwired: 1 out]
          n140 = Unbundle By Name(w368) -> ("X Array"=w370:dbl[], "Y Array"=w369:dbl[], "Original XY Plot Properties"=w361:T2)
          n141 = call "XY Graph Get-Set Plot Style.vi"("Error In"=w366, "Plot Index"=0, "XYGraph in"=w374) -> ("Error Out"=w364:errorcluster, "Plot Style out"=w365:T2)  [unwired: 5 in, 2 out]
          n142 = call "Get Notebook Queue.vi"() -> ("Notebook Queue"=w357:refnum<queue>)  [unwired: 9 in]
          n143 = Format Into String(format string="Plot %s edited:\n%s", w367, w356) -> (resulting string=w358:string)  [unwired: 2 in, 1 out]
          n144 = call "Restore X & Scale Indices.vi"("New Plot Style in"=w365, "Original Plot Style in"=w361) -> ("Updated Plot Style out"=w362:T2)  [unwired: 13 in]
          n145 = call "Message Style.vi"() -> ("Message Formatting"=w359:T8)
          n146 = call "Send Message to Notebook.vi"("Notebook Queue"=w357, "Message"=w358, "Text Formatting"=w359) -> ()  [unwired: 16 in, 1 out]
          n147 = call "XY Graph Update Plot & Style.vi"("Y Array"=w369, "X Array"=w370, "Error In"=w364, "XY Plot Properties"=w362, "Plot Idx"=w371, "XY Graph refnum"=w372) -> ()  [unwired: 5 in, 1 out]
        }
        frame "Copy & Quit" {
          n148 = Unbundle By Name(w403) -> ("VI title suffix"=w402:string)  [unwired: 1 out]
          n149 = Unbundle By Name(w403) -> ("X Array"=w391:dbl[], "Y Array"=w390:dbl[], "Original XY Plot Properties"=w388:T2)
          n150 = Unbundle By Name(w388) -> ("Plot.Plot Name"=w387:string)
          n151 = call "XY Graph Get-Set Plot Style.vi"("Error In"=w401, "Plot Index"=0, "XYGraph in"=w405) -> ("Error Out"=w398:errorcluster, "Plot Style out"=w400:T2)  [unwired: 5 in, 2 out]
          n152 = Concatenate Strings(w387, " (dup., edit.)" ("string")) -> (w392:string)
          n153 = call "Restore X & Scale Indices.vi"("New Plot Style in"=w400, "Original Plot Style in"=w388) -> ("Updated Plot Style out"=w395:T2)  [unwired: 13 in]
          n154 = Bundle("X Array"=w391, "Y Array"=w390) -> (w389:cluster{"X Array":dbl[], "Y Array":dbl[]})  [unwired: 1 in]
          n155 = call "XY Graph Add Single Plot with Name.vi"("XYGraph Ref in"=w396, "Plot"=w389, "Plot Name (\"Plot\")"=w392, "error in (no error)"=w398) -> ("Plot Index"=w394:i32, "Plot Name"=w380:string, "error out"=w382:errorcluster)  [unwired: 8 in, 1 out]
          n156 = Format Into String(format string="Copy Plot to %s\n", initial string=w386, error in=w382, w380) -> (resulting string=w379:string, error out=w377:errorcluster)
          n157 = call "Get Notebook Queue.vi"() -> ("Notebook Queue"=w383:refnum<queue>)  [unwired: 9 in]
          n158 = Format Into String(format string="Plot %s edited:%s", error in=w377, w402, w379) -> (resulting string=w384:string, error out=w376:errorcluster)  [unwired: 1 in]
          n159 = call "XY Graph Get-Set Plot Style.vi"("Error In"=w377, "Plot Index"=w394, "Plot Style in"=w395, "XYGraph in"=w396) -> ("Error Out"=w397:errorcluster)  [unwired: 4 in, 3 out]
          n160 = call "Message Style.vi"() -> ("Message Formatting"=w385:T8)
          n161 = call "Send Message to Notebook.vi"("Notebook Queue"=w383, "Message"=w384, "Error In"=w376, "Text Formatting"=w385) -> ()  [unwired: 15 in, 1 out]
        }
        frame "Save Plot" {
          w414 = T10 3 items=["no dialog", "OK message", "continue or stop message", "OK message + warnings", "continue/stop + warnings"] ("type of dialog (OK msg:1)")
          n162 = call "XY Graph Save Plot.vi"("Error In"=w416, "Plot Index"=0, "XYGraph Ref"=w417) -> ("Error Out"=w407:errorcluster, "File Path"=w409:path)  [unwired: 4 in, 3 out]
          n163 = Format Into String(format string="Plot saved to %s\n", initial string=w411, error in=w407, w409) -> (resulting string=w408:string, error out=w406:errorcluster)
          n164 = call <vilib>:"Simple Error Handler.vi"("type of dialog (OK msg:1)"=w414, "error in (no error)"=w406) -> ("error out"=w415:errorcluster)  [unwired: 3 in, 4 out]
          n165 = call <vilib>:"Clear Errors.vi"("error in (no error)"=w415) -> ("error out"=w413:errorcluster)  [unwired: 5 in, 1 out]
        }
        frame "Load Plot" {
          w435 = T10 3 items=["no dialog", "OK message", "continue or stop message", "OK message + warnings", "continue/stop + warnings"] ("type of dialog (OK msg:1)")
          w425 = 1 ("Max Number of Plot to Load (-1: All)")
          n166 = call "XY Graph Load Plot(s) Event.vi"("Max Number of Plot to Load (-1: All)"=w425, "Error In"=w437, "XYGraph Ref"=w429) -> ("Error Out"=w431:errorcluster, "Message"=w421:string, "File Path(s)"=w422:path[], "# Plots Added"=w433:i32[])  [unwired: 3 in, 2 out]
          n167 = Add Array Elements(numeric array=w433) -> (sum=w432:i32)
          n168 = Equal?(x=w432, y=w425) -> (x = y?=w428:bool)
          n169 = case shown="True" w428 {
            tunnel: w431 -> [w440 w449]
            tunnel: [w440 w446] -> w430
            tunnel: w429 -> [_ w445]
            tunnel: w427 -> [w441 w444]
            tunnel: [w441 w443] -> w426
            tunnel: w424 -> [w439 w453]
            tunnel: [w439 w452] -> w423
            tunnel: w422 -> [_ _]
            tunnel: w421 -> [_ w451]
            tunnel: w420 -> [_ w442]
            frame False {
            }
            frame True {
              # "removes previous plot & updates data"
              n170 = Format Into String(format string="%s\n", initial string=w453, error in=w449, w451) -> (resulting string=w452:string, error out=w450:errorcluster)
              n171 = call "XY Graph Delete Plot.vi"("Error In"=w450, "Plot Index"=0, "XYGraph Ref"=w445) -> ("Error Out"=w447:errorcluster)  [unwired: 5 in, 3 out]
              n172 = call "Plot Editor_Plot to Data & Controls.vi"("Control Refnums"=w442, "XYGraph in"=w445, "error in (no error)"=w447, "Plot Editor Internal Data in"=w444) -> ("error out"=w446:errorcluster, "Plot Editor Internal Data out"=w443:T6)  [unwired: 6 in]
            }
          }
          n173 = call <vilib>:"Simple Error Handler.vi"("type of dialog (OK msg:1)"=w435, "error in (no error)"=w430) -> ("error out"=w436:errorcluster)  [unwired: 3 in, 4 out]
          n174 = call <vilib>:"Clear Errors.vi"("error in (no error)"=w436) -> ("error out"=w434:errorcluster)  [unwired: 5 in, 1 out]
        }
        frame "Remove out-of-bound Values" {
          n175 = call "Plot Editor_Remove out-of-bound Plot Values.vi"("Control Refnums"=w455, "XYGraph in"=w460, "error in (no error)"=w466, "Plot Editor Internal Data"=w457) -> ("error out"=w462:errorcluster, "Message"=w459:string, "Plot Editor Internal Data out"=w456:T6)  [unwired: 5 in]
          n176 = Format Into String(format string="%s\n", initial string=w465, error in=w462, w459) -> (resulting string=w464:string, error out=w461:errorcluster)
        }
        frame "Delete Element", Default {
          n177 = Variant To Data(error in=w471, type=cluster{"CtlRef":refnum<vi>, "Coords":T7} {"CtlRef"=refnum, "Coords"={"Horizontal"=0, "Vertical"=0}} ("output cluster"), Variant=w486) -> (data=w484:cluster{"CtlRef":refnum<vi>, "Coords":T7}, error out=w477:errorcluster)
          n178 = Unbundle(w484) -> ("CtlRef"=w483:refnum<vi>, "Coords"=w482:T7)
          n179 = call "Determine Clicked Array Element Index.vi"("Error In"=w477, "Coords of Click"=w482, "Array Refnum"=w483) -> ("Error Out"=w478:errorcluster, "Clicked Row"=w481:i32)  [unwired: 1 in, 6 out]
          n180 = case shown="0, Default" w481 {
            selector: w481 -> [w498 _]
            tunnel: w480 -> [w507 _]
            tunnel: w479 -> [w506 _]
            tunnel: w478 -> [w500 w509]
            tunnel: w476 -> [w502 w511]
            tunnel: [w501 w511] -> w475
            tunnel: w474 -> [w496 w510]
            tunnel: [w496 w510] -> w473
            tunnel: [w490 w509] -> w472
            tunnel: w470 -> [w494 w508]
            tunnel: w469 -> [w487 _]
            tunnel: w468 -> [w492 _]
            tunnel: [w493 w508] -> w467
            frame 0, Default {
              w503 = 1 ("length")
              n181 = property class="Arr (strict)"(reference=w507, error in=w500) -> (error out=w497:errorcluster, "Value"=w505:dbl[])  [unwired: 1 out]
              n182 = property class="Arr (strict)"(reference=w506, error in=w500) -> (error out=w495:errorcluster, "Value"=w504:dbl[])  [unwired: 1 out]
              n183 = Format Into String(format string="Deleted element %d\n", initial string=w502, error in=w500, w498) -> (resulting string=w501:string)  [unwired: 1 out]
              n184 = Delete From Array(array=w505, length=w503, index=w498) -> (array with subset deleted=w489:dbl[])  [unwired: 1 out]
              n185 = Delete From Array(array=w504, length=w503, index=w498) -> (array with subset deleted=w488:dbl[])  [unwired: 1 out]
              n186 = Merge Errors(w497, w495) -> (w491:errorcluster)
              n187 = call "Plot Editor_Data to Controls & Plot.vi"("Plot Editor Internal Data"=w494, "XYGraph in"=w492, "X Array"=w489, "Y Array"=w488, "error in (no error)"=w491, "Control Refnums"=w487) -> ("Plot Editor Internal Data"=w493:T6, "error out"=w490:errorcluster)  [unwired: 8 in]
            }
            frame -1 {
            }
          }
        }
        frame "Insert Element Before" {
          n188 = Variant To Data(error in=w517, type=cluster{"CtlRef":refnum<vi>, "Coords":T7} {"CtlRef"=refnum, "Coords"={"Horizontal"=0, "Vertical"=0}} ("output cluster"), Variant=w531) -> (data=w529:cluster{"CtlRef":refnum<vi>, "Coords":T7}, error out=w522:errorcluster)
          n189 = Unbundle(w529) -> ("CtlRef"=w528:refnum<vi>, "Coords"=w527:T7)
          n190 = call "Determine Clicked Array Element Index.vi"("Error In"=w522, "Coords of Click"=w527, "Array Refnum"=w528) -> ("Error Out"=w523:errorcluster, "Clicked Row"=w526:i32)  [unwired: 1 in, 6 out]
          n191 = case shown="0, Default" w526 {
            selector: w526 -> [w545 _]
            tunnel: w525 -> [w552 _]
            tunnel: w524 -> [w551 _]
            tunnel: w523 -> [w543 w554]
            tunnel: w521 -> [w547 w556]
            tunnel: [w544 w556] -> w520
            tunnel: w519 -> [w542 w555]
            tunnel: [w542 w555] -> w518
            tunnel: [w536 w554] -> w516
            tunnel: w515 -> [w539 w553]
            tunnel: [w537 w553] -> w514
            tunnel: w513 -> [w538 _]
            tunnel: w512 -> [w532 _]
            frame 0, Default {
              w548 = nan ("new element/subarray")
              n192 = property class="Arr (strict)"(reference=w552, error in=w543) -> (error out=w541:errorcluster, "Value"=w550:dbl[])  [unwired: 1 out]
              n193 = property class="Arr (strict)"(reference=w551, error in=w543) -> (error out=w540:errorcluster, "Value"=w549:dbl[])  [unwired: 1 out]
              n194 = Insert Into Array(array=w550, index=w545, new element=w548) -> (w534:dbl[])
              n195 = Insert Into Array(array=w549, index=w545, new element=w548) -> (w533:dbl[])
              n196 = Format Into String(format string="Element inserted before %d\n", initial string=w547, error in=w543, w545) -> (resulting string=w544:string)  [unwired: 1 out]
              n197 = Merge Errors(w541, w540) -> (w535:errorcluster)
              n198 = call "Plot Editor_Data to Controls & Plot.vi"("Plot Editor Internal Data"=w539, "XYGraph in"=w538, "X Array"=w534, "Y Array"=w533, "error in (no error)"=w535, "Control Refnums"=w532) -> ("Plot Editor Internal Data"=w537:T6, "error out"=w536:errorcluster)  [unwired: 8 in]
            }
            frame -1 {
            }
          }
        }
        frame "Insert Element After" {
          n199 = Variant To Data(error in=w562, type=cluster{"CtlRef":refnum<vi>, "Coords":T7} {"CtlRef"=refnum, "Coords"={"Horizontal"=0, "Vertical"=0}} ("output cluster"), Variant=w576) -> (data=w574:cluster{"CtlRef":refnum<vi>, "Coords":T7}, error out=w569:errorcluster)
          n200 = Unbundle(w574) -> ("CtlRef"=w571:refnum<vi>, "Coords"=w570:T7)
          n201 = call "Determine Clicked Array Element Index.vi"("Error In"=w569, "Coords of Click"=w570, "Array Refnum"=w571) -> ("Error Out"=w568:errorcluster, "Clicked Row"=w567:i32)  [unwired: 1 in, 6 out]
          n202 = case shown="0, Default" w567 {
            selector: w567 -> [w594 _]
            tunnel: w573 -> [w598 _]
            tunnel: w572 -> [w597 _]
            tunnel: w568 -> [w589 w600]
            tunnel: w566 -> [w592 w602]
            tunnel: [w590 w602] -> w565
            tunnel: w564 -> [w580 w601]
            tunnel: [w580 w601] -> w563
            tunnel: [w582 w600] -> w561
            tunnel: w560 -> [w587 w599]
            tunnel: [w581 w599] -> w559
            tunnel: w558 -> [w577 _]
            tunnel: w557 -> [w578 _]
            frame 0, Default {
              w593 = nan ("new element/subarray")
              n203 = property class="Arr (strict)"(reference=w598, error in=w589) -> (error out=w585:errorcluster, "Value"=w596:dbl[])  [unwired: 1 out]
              n204 = property class="Arr (strict)"(reference=w597, error in=w589) -> (error out=w584:errorcluster, "Value"=w595:dbl[])  [unwired: 1 out]
              n205 = Increment(x=w594) -> (x+1=w588:i32)
              n206 = Insert Into Array(array=w596, index=w588, new element=w593) -> (w586:dbl[])
              n207 = Format Into String(format string="Element inserted after %d\n", initial string=w592, error in=w589, w588) -> (resulting string=w590:string)  [unwired: 1 out]
              n208 = Insert Into Array(array=w595, index=w588, new element=w593) -> (w579:dbl[])
              n209 = Merge Errors(w585, w584) -> (w583:errorcluster)
              n210 = call "Plot Editor_Data to Controls & Plot.vi"("Plot Editor Internal Data"=w587, "XYGraph in"=w578, "X Array"=w586, "Y Array"=w579, "error in (no error)"=w583, "Control Refnums"=w577) -> ("Plot Editor Internal Data"=w581:T6, "error out"=w582:errorcluster)  [unwired: 8 in]
            }
            frame -1 {
            }
          }
        }
        frame "Update output string" {
          n211 = call "Variant to String.vi"("Variant"=w610) -> ("String"=w604:string)  [unwired: 8 in]
          n212 = Format Into String(format string="%s\n", initial string=w609, error in=w605, w604) -> (resulting string=w608:string, error out=w606:errorcluster)
        }
        frame "Remove NaN-containing Pairs" {
          n213 = call "Variant to I32.vi"("Variant"=w627) -> ()  [unwired: 8 in, 1 out]
          n214 = Unbundle By Name(w615) -> ("X Array"=w626:dbl[], "Y Array"=w625:dbl[])
          n215 = call "Remove NaN-containing Pairs.vi"("Error In"=w621, "Y Array in"=w625, "X Array in"=w626) -> ("Error Out"=w620:errorcluster, "Y Array out"=w617:dbl[], "# X elts deleted"=w624:i32, "X Array out"=w618:dbl[])  [unwired: 5 in]
          n216 = case shown="1, Default" w624 {
            selector: w624 -> [_ w643]
            tunnel: [w630 w642] -> w622
            tunnel: w623 -> [w630 w640]
            tunnel: w620 -> [w629 w635]
            tunnel: [w629 w639] -> w619
            tunnel: w618 -> [_ w638]
            tunnel: w617 -> [_ w636]
            tunnel: w615 -> [w628 w637]
            tunnel: w614 -> [_ w634]
            tunnel: [w628 w633] -> w613
            tunnel: w612 -> [_ w632]
            frame 0 {
            }
            frame 1, Default {
              n217 = call "Plot Editor_Data to Controls & Plot.vi"("Plot Editor Internal Data"=w637, "XYGraph in"=w632, "X Array"=w638, "Y Array"=w636, "error in (no error)"=w635, "Control Refnums"=w634) -> ("Plot Editor Internal Data"=w633:T6, "error out"=w631:errorcluster)  [unwired: 8 in]
              n218 = Format Into String(format string="%d NaN-containing pair(s)  removed\n", initial string=w640, error in=w631, w643) -> (resulting string=w642:string, error out=w639:errorcluster)
            }
          }
        }
        frame "Fill Array with Ramp" {
          n219 = call-by-ref "?"("error in (no error)"=w654) -> ("error out"=w648:errorcluster, "OK?"=w653:bool, "Ramp"=w652:dbl[])  [unwired: 10 in, 2 out]
          n220 = case shown="True" w653 {
            tunnel: w656 -> [w660 w679]
            tunnel: [w660 w668] -> w655
            tunnel: w652 -> [_ w674]
            tunnel: w651 -> [w659 w678]
            tunnel: [w659 w677] -> w650
            tunnel: w649 -> [w658 w667]
            tunnel: w648 -> [w657 w666]
            tunnel: [w657 w663] -> w647
            tunnel: [w658 w667] -> w646
            tunnel: w645 -> [_ w662]
            tunnel: w644 -> [_ w661]
            frame False {
            }
            frame True {
              n221 = Array Size(array=w674) -> (size(s)=w673:i32)
              n222 = Decrement(x=w673) -> (x-1=w672:i32)
              n223 = Bundle By Name(cluster=w679, "X Array"=w674) -> (w670:T6)
              n224 = Index Array(array=w674, index #2=w672) -> (element #1=w675:dbl, element #2=w671:dbl)  [unwired: 1 in]
              n225 = call "Plot Editor_Store to Controls.vi"("Error In"=w666, "Control Refnums"=w662, "Plot Editor Internal Data in"=w670) -> ("Error Out"=w665:errorcluster, "Plot Editor Internal Data out"=w669:T6)  [unwired: 7 in]
              n226 = call "Plot Editor_Store to Plot.vi"("XYGraph in"=w661, "Error In"=w665, "Plot Editor Internal Data"=w669) -> ("Error Out"=w664:errorcluster, "Plot Editor Internal Data (dup)"=w668:T6)  [unwired: 7 in]
              n227 = Format Into String(format string="X array filled with ram (%#g...%#g [%d])\n", initial string=w678, error in=w664, w675, w671, w673) -> (resulting string=w677:string, error out=w663:errorcluster)
            }
          }
        }
        frame "Quit" {
          n228 = Unbundle By Name(w685) -> ("Original X Array"=w684:dbl[], "Original Y Array"=w683:dbl[], "Original XY Plot Properties"=w682:T2)
          n229 = Bundle By Name(cluster=w685, "X Array"=w684, "Y Array"=w683) -> (w686:T6)
        }
      }
      n230 = Empty Array?(array=w254) -> (empty?=w253:bool)
    }
    "Error" <- w217
  }
  "Plot Style out" <- w28
  "Error Out" <- w33
  n231 = Unregister For Events(event registration refnum=w23) -> ()  [unwired: 1 in, 1 out]
  n232 = Unbundle By Name(w32) -> ("Refnum based call"=w17:bool, "X Array"=w31:dbl[], "Y Array"=w30:dbl[])
  n233 = Release Queue(queue=w38) -> ()  [unwired: 2 in, 3 out]
  n234 = invoke class="VI" method="FP.Close"(reference=w18) -> (reference out=w15:refnum<vi>, error out=w11:errorcluster)  [unwired: 2 in, 1 out]
  n235 = case shown="False" w17 {
    tunnel: w15 -> [w689 w693]
    tunnel: [w689 w692] -> w14
    tunnel: [w688 w691] -> w12
    tunnel: w11 -> [w688 w690]
    frame False {
    }
    frame True {
      n236 = invoke class="VI" method="Abort VI"(reference=w693, error in=w690) -> (reference out=w692:refnum<vi>, error out=w691:errorcluster)  [unwired: 1 in, 1 out]
    }
  }
  n237 = Bundle("X Array"=w31, "Y Array"=w30) -> (→"Plot out":cluster{"X Array":dbl[], "Y Array":dbl[]})  [unwired: 1 in]
  n238 = Close Reference(reference=w14, error in (no error)=w12) -> (error out=w13:errorcluster)
  n239 = call "Clear Error.vi"("Error In"=w13) -> ()  [unwired: 8 in, 1 out]
